vi "Decimate waveform.vi"(0 "reference in":refnum<class "Fcurve.lvclass">, 2 "Segment zeroed fcurve data":cluster{"X":dbl[], "Y":dbl[]}[](array[cluster]), 5 "error in (no error)":errorcluster) -> (14 "reference out":refnum<class "Fcurve.lvclass">, 15 "Decimated Fcurve (App,Con,Ret)":cluster{"X":dbl[], "Y":dbl[]}[](array[cluster]), 19 "error out":errorcluster)   [LabVIEW 2019, in "Fcurve.lvclass"]
doc: "Gets the waveforms and decimates them by a chosen decimating factor"
uses:
  Fcurve.lvclass
  <vilib>/Analysis/2dsp.llb/Decimate (single shot, DBL).vi
  <vilib>/Analysis/NI_AALPro.lvlib
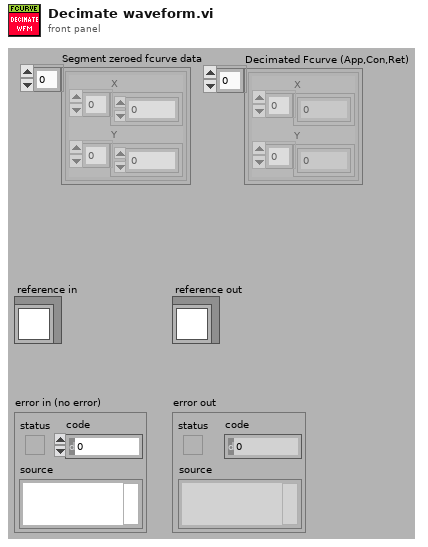
[diagram p1: front panel]
types:
  T1 = typedef "Fcurve.lvclass/ObjectAttributes.ctl" = cluster{"MyAttribute":dbl, "Fcurve Metadata":T2, "Contact Spread of dev":dbl, "Tau Delay (ms)":dbl, "Points of contact":dbl, "Def_wfm":cluster{"Max":dbl, "Min":dbl}, "Zpos_wfm":cluster{"Max":dbl, "Min":dbl}, "Contact stat?":bool, "Real AI dt (s)":dbl, "Decimation":cluster{"App":cluster{"Dec":i32, "apply":bool}, "Con":cluster{"Dec":i32, "apply":bool}, "Ret":cluster{"Dec":i32, "apply":bool}}, "Segment def[0]":dbl, "Segment Zpos[0]":dbl, "Raw Datum":waveform(dbl)[], "Group metadata":T3, "M_data obj":refnum<class "metadata.lvclass">, "Channel name(s)":string[], "Segment fcurve data":cluster{"X":dbl[], "Y":dbl[]}[], "Segment duration":cluster{"Start":i32, "Duration":i32}[], "Segment info":T4[], "Segment durations (S)":dbl[], "Segments Maxmin":T6[]}
  T2 = typedef "Fcurve.lvclass/Metadata.ctl" = cluster{"dt (us)":dbl, "Dec Factor":dbl, "Z piezo Sensitivity (nm/V)":dbl, "K (N/m)":dbl, "Sp (V)":dbl, "Contact (ms)":dbl, "Zpos contact":dbl, "Vel_app (nm/s)":dbl, "Vel_ret (nm/s)":dbl, "deltaV (nm)":dbl, "Def_V0 (v)":dbl, "Piezo gain":dbl, "invOLS (nm/V)":dbl}
  T3 = typedef "TDMS_DataHandler.lvclass/Fcurve Meta data.ctl" = cluster{"property names":string[], "property values":variant[]}
  T4 = typedef "Fcurve.lvclass/Fcurve segments --cluster.ctl" = cluster{"type":T5, "nb points":i32, "dec factor":u32, "sampling rate (S/s)":u32}
  T5 = typedef "metadata.lvclass/Segment type--combobox.ctl" = string
  T6 = typedef "Fcurve.lvclass/Segment MaxMin --cluster.ctl" = cluster{"Def":cluster{"max value":dbl, "min value":dbl}, "Zpos":cluster{"max value":dbl, "min value":dbl}}
  T7 = cluster{"App":cluster{"Dec":i32, "apply":bool}, "Con":cluster{"Dec":i32, "apply":bool}, "Ret":cluster{"Dec":i32, "apply":bool}}
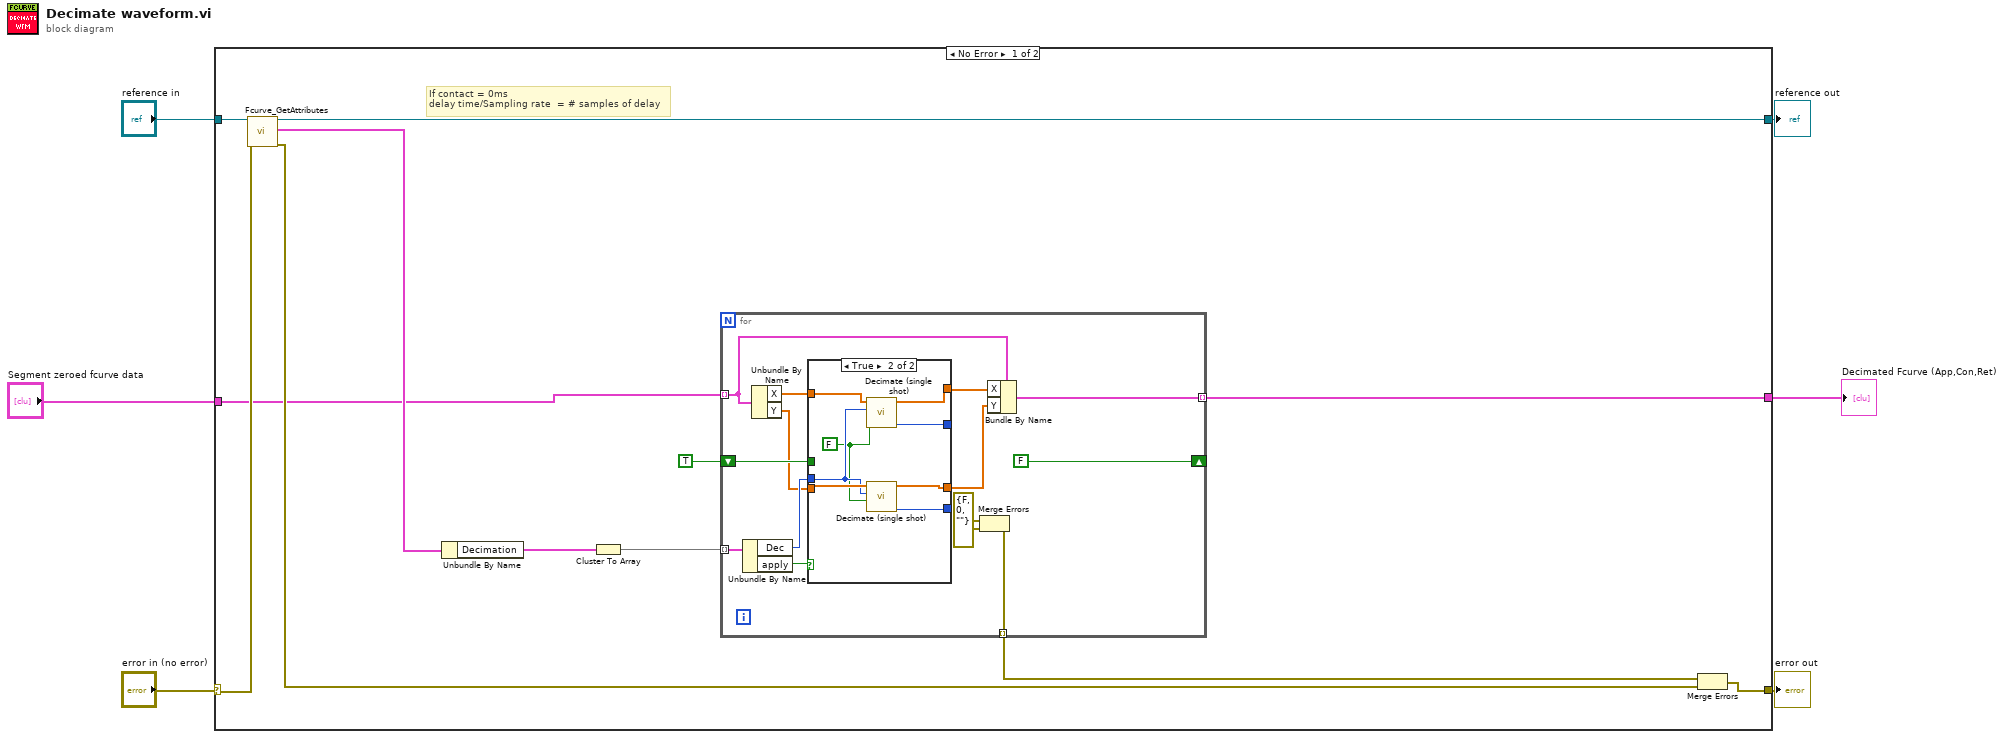
[diagram p0: block diagram]
diagram:
  n1 = case shown="No Error" "error in (no error)" {
    selector: "error in (no error)" -> [w16 w43]
    tunnel: [w18 w43] -> w5
    tunnel: [w17 w42] -> w3
    tunnel: "reference in" -> [w14 w42]
    tunnel: [w8 _] -> w2
    tunnel: "Segment zeroed fcurve data" -> [w7 _]
    frame No Error {
      # "If contact = 0ms\ndelay time/Sampling rate  = # samples of delay"
      n2 = call "Fcurve_GetAttributes.vi"("reference in"=w14, "error in (no error)"=w16) -> ("reference out"=w17:refnum<class "Fcurve.lvclass">, "attributes"=w15:T1, "error out"=w13:errorcluster)  [unwired: 14 in, 1 out]
      n3 = Unbundle By Name(w15) -> ("Decimation"=w12:T7)
      n4 = Cluster To Array(cluster=w12) -> (array=w11:cluster{"Dec":i32, "apply":bool}[])
      n5 = for {
        tunnel: w7 -> [w31] mode=indexing
        tunnel: w11 -> [w30] mode=indexing
        shift-right: [FALSE ("reset")] -> _
        shift-left: TRUE ("reset") -> [w27]
        tunnel: [w21] -> w9 mode=indexing
        tunnel: [w20] -> w8 mode=indexing
        w19 = errorcluster {"status"=FALSE, "code"=0, "source"=""} ("error in")
        n6 = Unbundle By Name(w30) -> ("Dec"=w29:i32, "apply"=w26:bool)
        n7 = Unbundle By Name(w31) -> ("X"=w25:dbl[], "Y"=w24:dbl[])
        n8 = case shown="True" w26 {
          tunnel: w29 -> [_ w37]
          tunnel: w27 -> [_ _]
          tunnel: w25 -> [w33 w41]
          tunnel: w24 -> [w32 w38]
          tunnel: [w33 w40] -> w23
          tunnel: [w32 w35] -> w22
          tunnel: [_ w39] -> _
          tunnel: [_ w34] -> _
          frame False {
          }
          frame True {
            w36 = FALSE ("averaging")
            n9 = call-poly <vilib>:"Decimate (single shot).vi"("averaging"=w36, "decimating factor"=w37, "X"=w41) -> ("error"=w39:i32, "Decimated Array"=w40:dbl[])  [unwired: 7 in]
            n10 = call-poly <vilib>:"Decimate (single shot).vi"("averaging"=w36, "decimating factor"=w37, "X"=w38) -> ("error"=w34:i32, "Decimated Array"=w35:dbl[])  [unwired: 7 in]
          }
        }
        n11 = Merge Errors(w19, w19) -> (w21:errorcluster)
        n12 = Bundle By Name(cluster=w31, "X"=w23, "Y"=w22) -> (w20:cluster{"X":dbl[], "Y":dbl[]})
      }
      n13 = Merge Errors(w9, w13) -> (w18:errorcluster)
    }
    frame Error {
    }
  }
  "error out" <- w5
  "reference out" <- w3
  "Decimated Fcurve (App,Con,Ret)" <- w2
